vi "audio filter.vi"(3 "audio off state (V)":dbl, 4 "audio filter period(uSec)":i32, 5 "audio threshold":fxp<+/-,16,5>, 6 "input":dbl) -> (2 "output":bool)   [LabVIEW 2014]
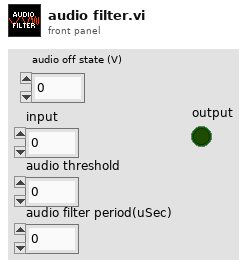
[diagram p1: front panel]
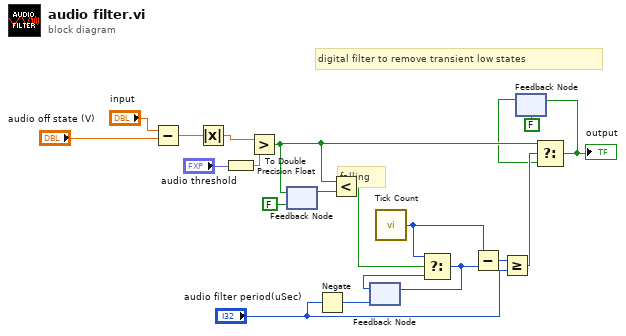
[diagram p0: block diagram]
diagram:
  # "digital filter to remove transient low states"
  # "falling"
  n1 = Subtract(x="input", y="audio off state (V)") -> (x-y=w1:dbl)
  n2 = Absolute Value(x=w1) -> (abs(x)=w2:dbl)
  n3 = To Double Precision Float(number="audio threshold") -> (double precision float=w5:dbl)
  n4 = Greater?(x=w2, y=w5) -> (0:w16:bool)
  n5 = feedback #1(FALSE) -> (w15:bool)
  n6 = feedback-in #1(w16) -> ()
  n7 = Negate(x="audio filter period(uSec)") -> (-x=w10:i32)
  n8 = Less?(x=w16, y=w15) -> (x < y?=w20:bool)
  n9 = feedback #2(w10) -> (w12:u32)
  n10 = call "Tick Count"() -> ("Tick Count(uSec)"=w19:u32)
  n11 = Select(t=w19, s=w20, f=w12) -> (s? t:f=w13:u32)
  n12 = feedback-in #2(w13) -> ()
  n13 = Subtract(x=w19, y=w13) -> (x-y=w18:u32)
  n14 = Greater Or Equal?(x=w18, y="audio filter period(uSec)") -> (x >= y?=w17:bool)
  n15 = feedback #3(FALSE) -> (w8:bool)
  n16 = Select(t=w16, s=w17, f=w8) -> (s? t:f=w9:bool)
  "output" <- w9
  n17 = feedback-in #3(w9) -> ()
